vi "Save Configuration.vi"(8 "error in (no error)":errorcluster, 10 "File path":path, 11 "Monitor-Pulse in":refnum<class "Monitor-Pulse.lvclass">) -> (0 "error out":errorcluster, 1 "Section out":string, 2 "File path out":path, 3 "Monitor-Pulse out":refnum<class "Monitor-Pulse.lvclass">)   [LabVIEW 2016, in "Monitor-Pulse.lvclass"]
uses:
  Monitor-Pulse.lvclass
  D:/github/Measure_core/Measure Object/Measure Object.lvclass
  Measure_core/Measure Object/Measure Object.lvclass/Measure Object.ctl
  Monitor-Pulse.lvclass/Monitor-Pulse.ctl
  NHMFL_Core/Libraries/Queued Listbox/Queued Listbox.xctl
  Measure_core/Measure Object/Read Name.vi
  Measure_core/Controllers/Process Controller/Process Controller.lvclass
  <vilib>/Utility/config.llb/NI_LVConfig.lvlib
panel:
  out "Array":string[](array[string])
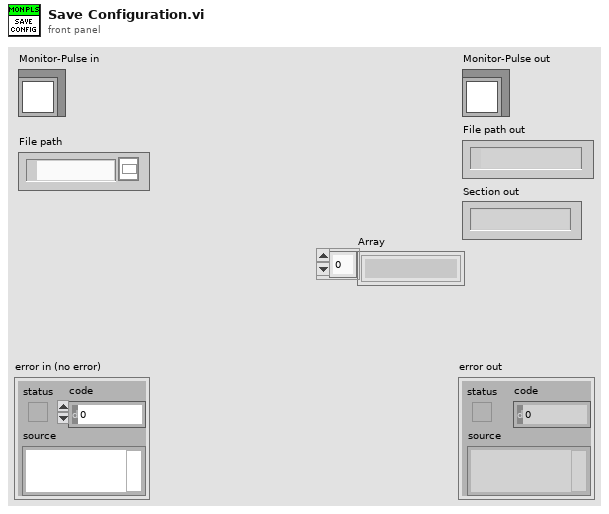
[diagram p1: front panel]
types:
  T1 = typedef "NI_LVConfig.lvlib/Config Data RefNum.ctl" = refnum<k1>
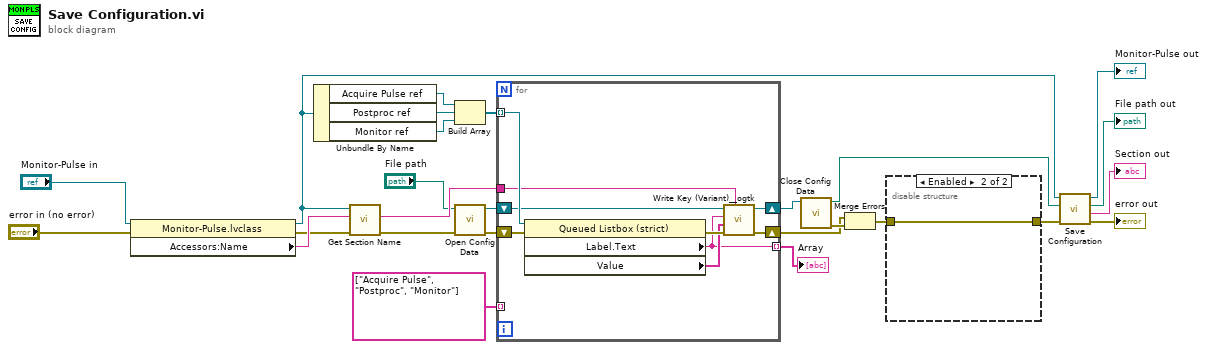
[diagram p0: block diagram]
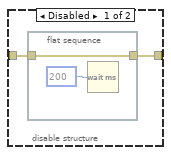
[diagram p2: hidden frame]
diagram:
  n1 = property class="Monitor-Pulse.lvclass"(reference="Monitor-Pulse in", error in="error in (no error)") -> (reference out=w8:refnum<class "Monitor-Pulse.lvclass">, error out=w1:errorcluster, "Accessors:Name"=w14:string)
  n2 = Unbundle By Name(w8) -> ("Acquire Pulse ref"=w26:refnum<vi>, "Postproc ref"=w25:refnum<vi>, "Monitor ref"=w24:refnum<vi>)
  n3 = call "Get Section Name.vi"("Error In"=w1, "Object name"=w14, "object"=w8) -> ("Error Out"=w6:errorcluster, "Section out"=w13:string)  [unwired: 7 in]
  n4 = Build Array(w26, w25, w24) -> (w23:refnum<vi>[])
  n5 = call <vilib>:"Open Config Data.vi"("error in (no error)"=w6, "configuration file path"="File path") -> ("error out"=w5:errorcluster, "refnum"=w22:T1)  [unwired: 7 in, 1 out]
  n6 = for {
    tunnel: w23 -> [w35] mode=indexing
    shift-right: [w30] -> w20
    shift-left: w5 -> [w34]
    shift-right: [w32] -> w19
    shift-left: w22 -> [w33]
    tunnel: w13 -> [w29]
    tunnel: string[] ["Acquire Pulse", "Postproc", "Monitor"] -> [_] mode=indexing
    tunnel: [w27] -> w16 mode=indexing
    n7 = property class="Queued Listbox (strict)"(reference=w35, error in=w34) -> (error out=w31:errorcluster, "Label.Text"=w27:string, "Value"=w28:string[])  [unwired: 1 out]
    n8 = call <userlib>:"Write Key (Variant)__ogtk.vi"("section"=w29, "error in (no error)"=w31, "key-value"=w28, "key (optional)"=w27, "refnum"=w33) -> ("error out"=w30:errorcluster, "refnum out"=w32:T1)  [unwired: 5 in]
  }
  "Array" <- w16
  n9 = call <vilib>:"Close Config Data.vi"("refnum"=w19) -> ("error out"=w21:errorcluster, "file path"=w11:path)  [unwired: 9 in]
  n10 = Merge Errors(w20, w21) -> (w10:errorcluster)
  n11 = disable-structure shown="Enabled" {
    disable-tunnel: w10 -> [w37 w40]
    disable-tunnel: [w36 w40] -> w9
    frame Disabled {
      n12 = flat-sequence {
        tunnel: w37 -> [w39]
        tunnel: [w39] -> w36
        frame #0 {
          n13 = Wait (ms)(milliseconds to wait=u32 200) -> ()  [unwired: 1 out]
        }
      }
    }
    frame Enabled {
    }
  }
  n14 = call-parent "Save Configuration.vi"("error in (no error)"=w9, "File path"=w11, "Measure Object in"=w8) -> ("error out"=→"error out":errorcluster, "Section out"=→"Section out":string, "File path out"=→"File path out":path, "Measure Object out"=→"Monitor-Pulse out":refnum<class "Monitor-Pulse.lvclass">)  [unwired: 5 in]
